vi "client.add.vi"(8 "error in (no error)":errorcluster, 9 "y":dbl, 11 "x":dbl) -> (0 "error out":errorcluster, 2 "x+y":dbl)   [LabVIEW 2016]
uses:
  <vilib>/NI/JSON Support for LabVIEW/JSON Value/New JSON Value/New JSON (Numeric[]).vi
  <vilib>/NI/NI JSONRPC Server Framework/Classes/Client/Format Client Request (Auto-Increment).vi
  <vilib>/httpClient/POSTBuffer.vi
  <vilib>/NI/JSON Support for LabVIEW/JSON Value/Read Value/Read value (Numeric).vi
  <vilib>/NI/JSON Support for LabVIEW/JSON Value/JSON Value.lvclass
  <vilib>/NI/NI JSONRPC Server Framework/Classes/Client/JSONRPC Client.lvclass
  <vilib>/httpClient/LabVIEWHTTPClient.lvlib
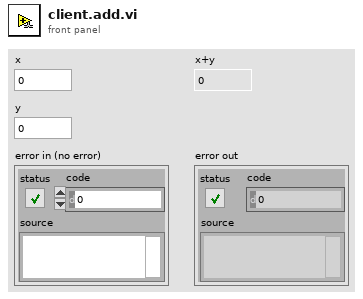
[diagram p1: front panel]
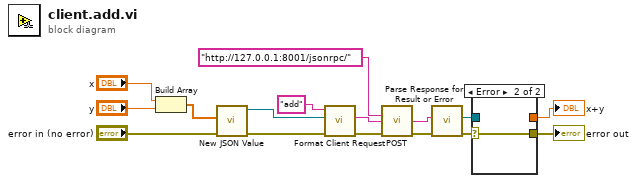
[diagram p0: block diagram]
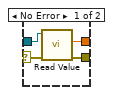
[diagram p2: hidden frame]
diagram:
  n1 = Build Array("x", "y") -> (w14:dbl[])
  n2 = call-poly <vilib>:"New JSON Value.vi"("error in (no error)"="error in (no error)", "Numeric Array"=w14) -> ("error out"=w11:errorcluster, "JSON Value out"=w12:refnum<class "JSON Value.lvclass">)  [unwired: 8 in]
  n3 = call-poly <vilib>:"Format Client Request.vi"("error in (no error)"=w11, "JSON Value in"=w12, "method"="add") -> ("error out"=w2:errorcluster, "Request String"=w4:string)  [unwired: 7 in]
  n4 = call-poly <vilib>:"POST.vi"("url"="http://127.0.0.1:8001/jsonrpc/", "buffer"=w4, "error in (no error)"=w2) -> ("body"=w3:string, "error out"=w1:errorcluster)  [unwired: 9 in, 2 out]
  n5 = call <vilib>:"Parse Response for Result or Error.vi"("error in"=w1, "Response String In"=w3) -> ("error out"=w9:errorcluster, "JSON Value out"=w8:refnum<class "JSON Value.lvclass">)  [unwired: 7 in, 1 out]
  n6 = case shown="Error" w9 {
    selector: w9 -> [w20 w21]
    tunnel: w8 -> [w19 _]
    tunnel: [w18 _] -> w7
    tunnel: [w17 w21] -> w6
    frame No Error {
      n7 = call-poly <vilib>:"Read Value.vi"("error in (no error)"=w20, "JSON Numeric in"=w19) -> ("error out"=w17:errorcluster, "value"=w18:dbl)  [unwired: 7 in, 1 out]
    }
    frame Error {
    }
  }
  "x+y" <- w7
  "error out" <- w6
